vi "niTuner Get Cal (single).vi"(8 "error in":errorcluster, 9 "correct for attenuation":bool=TRUE, 11 "taskID in":i32 format="%.0x") -> (0 "error out":errorcluster, 2 "calibration":T1(array[cluster]) {"array" format="%.2f"; "f2" format="%.2f"; "f1" format="%.2f"}, 3 "taskID out":i32 format="%.0x")   [LabVIEW 2011]
doc: "This VI returns calibration information for a single frequency entry in the scan list. The VI returns RF calibration information, IF calibration information, and (if correct for attenuation is set to TRUE) total attenuation calibration information."
uses:
  nipxi5600u.dll
  nidaq32.dll
panel:
  out "YIG tuned frequency":dbl format="%.2f"
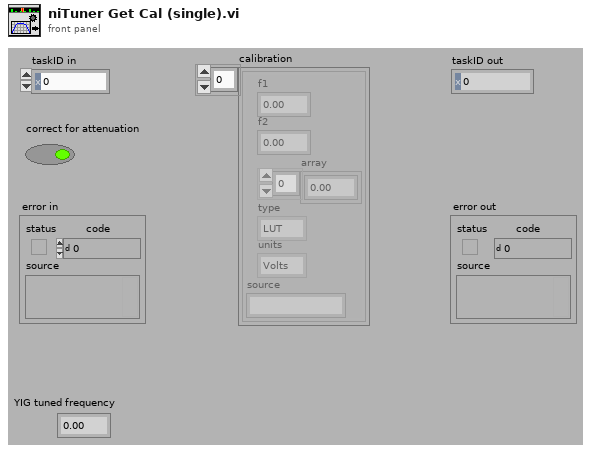
[diagram p1: front panel]
types:
  T1 = cluster{"f1":dbl, "f2":dbl, "array":sgl[], "type":enum16{"LUT", "polynomial"}, "units":enum16{"Volts", "Watts", "dBm", "dBW", "dBV", "dBmV", "dBuV"}, "source":string}[]
  T2 = cluster{"f1":dbl, "f2":dbl, "array":sgl[], "type":enum16{"LUT", "polynomial"}, "units":enum16{"Volts", "Watts", "dBm", "dBW", "dBV", "dBmV", "dBuV"}, "source":string}
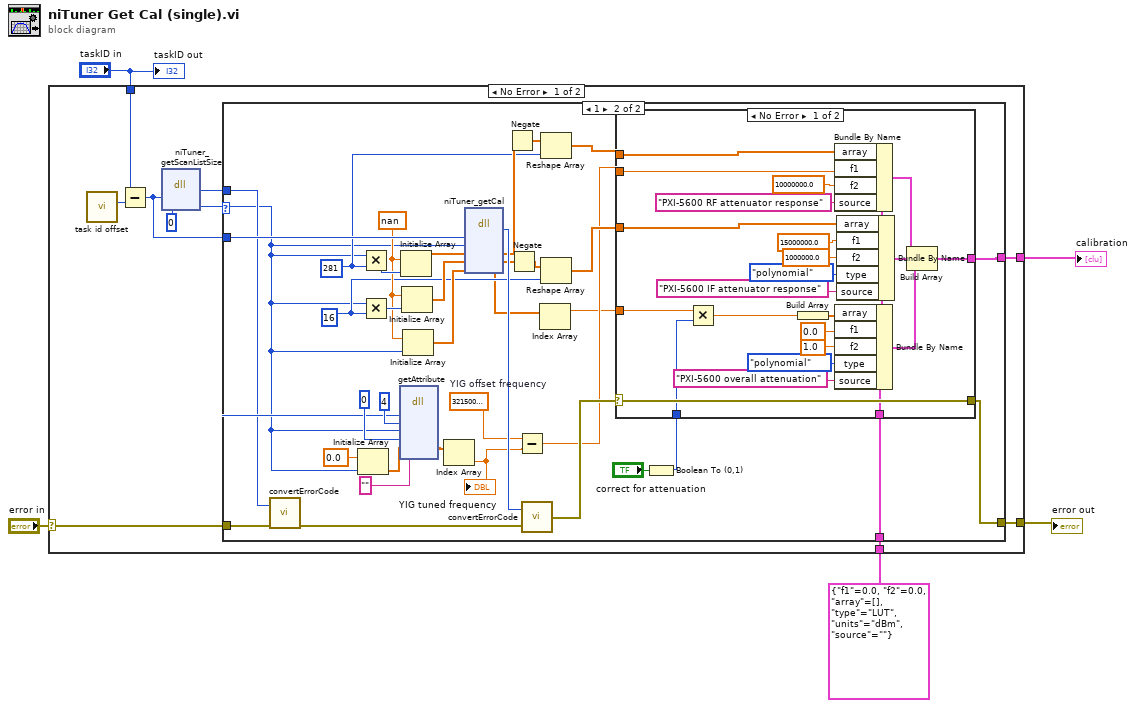
[diagram p0: block diagram]
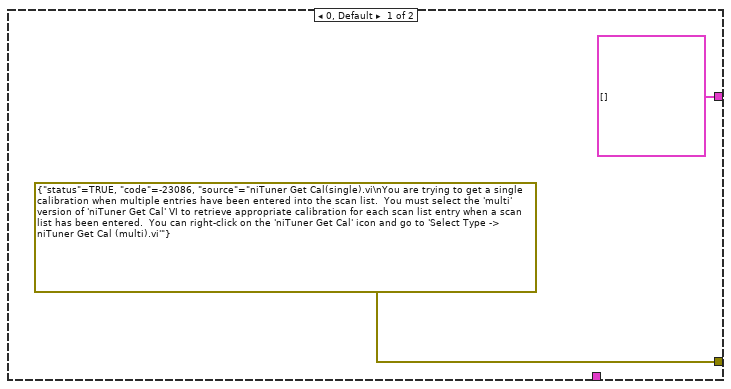
[diagram p2: hidden frame]
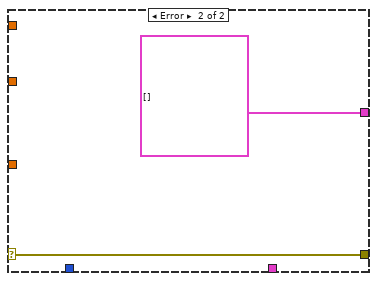
[diagram p3: hidden frame]
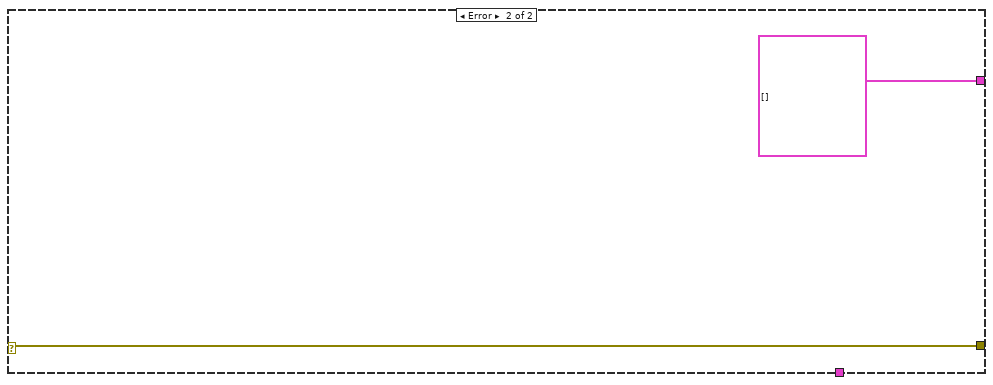
[diagram p4: hidden frame]
diagram:
  n1 = case shown="No Error" "error in" {
    selector: "error in" -> [w8 w81]
    tunnel: T2 {"f1"=0.0, "f2"=0.0, "array"=[], "type"=enum."LUT", "units"=enum."dBm", "source"=""} -> [w14 _]
    tunnel: [w13 w81] -> w3
    tunnel: "taskID in" -> [w12 _]
    tunnel: [w7 T1 []] -> w1
    frame No Error {
      n2 = call <instrlib>:"task id offset.vi"() -> ("taskID offset"=w15:i32)
      n3 = Subtract(x=w12, y=w15) -> (x-y=w10:i32)
      n4 = dll-call lib="nipxi5600u.dll" fn="niTuner_getScanListSize"("taskID"=w10, "scanListSize"=u32 0) -> (w9:i32, "scanListSize"=w6:u32)  [unwired: 4 in, 2 out]
      n5 = case shown="1" w6 {
        selector: w6 -> [_ w18]
        tunnel: w14 -> [_ w53]
        tunnel: [errorcluster {"status"=TRUE, "code"=-23086, "source"="niTuner Get Cal(single).vi\nYou are trying to get a single calibration when multiple entries have been entered into the scan list.  You must select the 'multi' version of 'niTuner Get Cal' VI to retrieve appropriate calibration for each scan list entry when a scan list has been entered.  You can right-click on the 'niTuner Get Cal' icon and go to 'Select Type -> niTuner Get Cal (multi).vi'"} ("error in 1 (no error)") w52] -> w13
        tunnel: w10 -> [_ w45]
        tunnel: w9 -> [_ w37]
        tunnel: w8 -> [_ w36]
        tunnel: [T1 [] w27] -> w7
        frame 0, Default {
        }
        frame 1 {
          w29 = 3215000000.0  # YIG offset frequency
          w31 = u32 16
          w41 = nan ("Element Data")
          w33 = u32 281
          n6 = call <instrlib>:"convertErrorCode.vi"("error in"=w36, "error code"=w37) -> ("error out"=w35:errorcluster)
          n7 = Initialize Array(0.0 ("Element Data"), w18) -> (w50:dbl[])
          n8 = Multiply(x=w18, y=w33) -> (x*y=w43:u32)
          n9 = Multiply(x=w18, y=w31) -> (x*y=w42:u32)
          n10 = dll-call lib="nidaq32.dll" fn="getAttribute"("device"=w45, "attribute"=u32 4, "u32val"=w18, "i32val"=0, "f64val"=w50, "strval"="") -> ("f64val"=w22:dbl[])  [unwired: 9 in, 2 out]
          n11 = Initialize Array(w41, w43) -> (w44:dbl[])
          n12 = Initialize Array(w41, w42) -> (w40:dbl[])
          n13 = Initialize Array(w41, w18) -> (w39:dbl[])
          n14 = Index Array(array=w22) -> (element=w21:dbl)  [unwired: 1 in]
          "YIG tuned frequency" <- w21
          n15 = dll-call lib="nipxi5600u.dll" fn="niTuner_getCal"("taskID"=w45, "listSize"=w18, "RFArrays"=w44, "IFArrays"=w40, "attenuationArray"=w39) -> (w54:i32, "RFArrays"=w38:dbl[], "IFArrays"=w32:dbl[], "attenuationArray"=w20:dbl[])  [unwired: 5 in, 2 out]
          n16 = Negate(x=w38) -> (-x=w24:dbl[])
          n17 = Negate(x=w32) -> (-x=w23:dbl[])
          n18 = Subtract(x=w29, y=w21) -> (x-y=w28:dbl)
          n19 = call <instrlib>:"convertErrorCode.vi"("error in"=w35, "error code"=w54) -> ("error out"=w34:errorcluster)
          n20 = Index Array(array=w20) -> (element=w19:dbl)  [unwired: 1 in]
          n21 = Reshape Array(w24, w33) -> (w51:dbl[])
          n22 = Reshape Array(w23, w31) -> (w30:dbl[])
          n23 = Boolean To (0,1)(Boolean="correct for attenuation") -> (0, 1=w25:i16)
          n24 = case shown="No Error" w34 {
            selector: w34 -> [w76 w79]
            tunnel: w51 -> [w77 _]
            tunnel: w53 -> [w72 _]
            tunnel: [w76 w79] -> w52
            tunnel: w28 -> [w75 _]
            tunnel: w30 -> [w74 _]
            tunnel: w19 -> [w73 _]
            tunnel: [w71 T1 []] -> w27
            tunnel: w25 -> [w70 _]
            frame No Error {
              n25 = Multiply(x=w73, y=w70) -> (x*y=w55:dbl)
              n26 = Build Array(w55) -> (w63:dbl[])
              n27 = Bundle By Name(cluster=w72, "array"=w77, "f1"=w75, "f2"=10000000.0, "source"="PXI-5600 RF attenuator response") -> (w58:T2)
              n28 = Bundle By Name(cluster=w72, "array"=w63, "f1"=0.0, "f2"=1.0, "type"=enum16{"LUT", "polynomial"}."polynomial", "source"="PXI-5600 overall attenuation") -> (w57:T2)
              n29 = Bundle By Name(cluster=w72, "array"=w74, "f1"=15000000.0, "f2"=1000000.0, "type"=enum16{"LUT", "polynomial"}."polynomial", "source"="PXI-5600 IF attenuator response") -> (w59:T2)
              n30 = Build Array(w58, w59, w57) -> (w71:T1)
            }
            frame Error {
            }
          }
        }
      }
    }
    frame Error {
    }
  }
  "calibration" <- w1
  "error out" <- w3
  "taskID out" <- "taskID in"
